vi "UnMangle VI Name__ogtk.vi"   [LabVIEW 2011]
doc: "Unmangles a VI's name by removing a <b>namespace string suffix</b>.\n<b>Name</b> may be a path or a string.\nFor example:\n\nMangled Name => \"Widget__OpenG.vi\"\nUnmangled Name => \"Widget.vi\"\nNamespace => \"OpenG\"\n\nMangled Name => \"Widget__OpenG\"\nUnmangled Name => \"Widget\"\nNamespace => \"OpenG\"\n\nMangled Name => \"Widget.vi\"\nUnmangled Name => \"Widget.vi\"\nNamespace => \"\" (Note: blank string means do not mangle)"
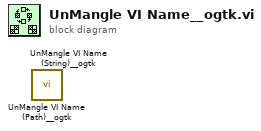
[diagram p0: block diagram]
diagram:
  n1 = call "UnMangle VI Name (Path)__ogtk.vi"() -> ()  [unwired: 9 in, 3 out]
  n2 = call "UnMangle VI Name (String)__ogtk.vi"() -> ()  [unwired: 9 in, 3 out]
